vi "get Settings.vi"() -> (3 "Settings":T1)   [LabVIEW 2015, in "System Config.lvclass"]
uses:
  System Config.lvclass
  protected/Settings.ctl
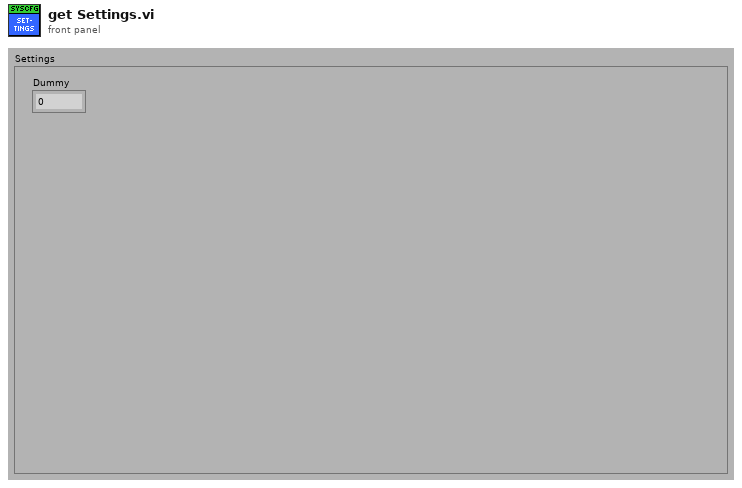
[diagram p1: front panel]
types:
  T1 = typedef "System Config.lvclass/Settings.ctl" = cluster{"Dummy":dbl}
  T2 = typedef "System Config.lvclass/ClassAttributes.ctl" = cluster{"Config":cluster{"Logging":cluster{"Log Files Directory":path, "Max Lines Per Log File":i32}, "Settings":T1}, "Core":cluster{"Config Directory":path, "Name":string, "Config Changed":refnum<user-event>}}
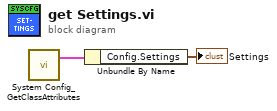
[diagram p0: block diagram]
diagram:
  n1 = call "System Config_GetClassAttributes.vi"() -> ("class attributes"=w2:T2)  [unwired: 8 in, 3 out]
  n2 = Unbundle By Name(w2) -> ("Config.Settings"=→"Settings":T1)
